vi "Control_stack_solenoid_top.vi"(0 "Valve On?":bool) -> (2 "s? t:f":errorcluster)   [LabVIEW 2010]
panel:
  in  "Reset":bool
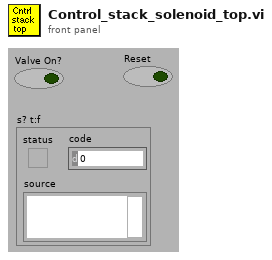
[diagram p1: front panel]
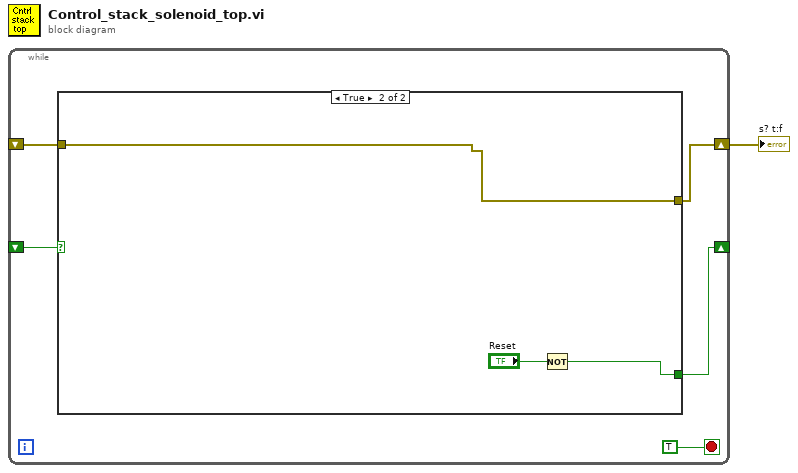
[diagram p0: block diagram]
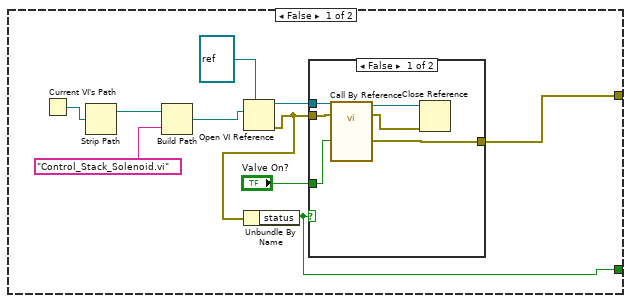
[diagram p2: hidden frame]
diagram:
  n1 = while {
    shift-right: [w5] -> _
    shift-left: _ -> [w6]
    shift-right: [w3] -> w1
    shift-left: _ -> [w2]
    stop <- TRUE stop-if-true
    n2 = case shown="True" w6 {
      tunnel: [w8 w24] -> w5
      tunnel: [w7 w26] -> w3
      tunnel: w2 -> [_ w26]
      frame False {
        n3 = Current VI's Path() -> (path=w16:path)
        n4 = Strip Path(path=w16) -> (stripped path=w15:path)  [unwired: 1 out]
        n5 = Build Path(base path=w15, name or relative path="Control_Stack_Solenoid.vi") -> (appended path=w13:path)
        n6 = Open VI Reference(type specifier VI Refnum (for type only)=refnum<vi> refnum, vi path=w13) -> (vi reference=w11:refnum<vi>, error out=w10:errorcluster)  [unwired: 1 in, 3 out]
        n7 = Unbundle By Name(w10) -> ("status"=w8:bool)
        n8 = case shown="False" w8 {
          tunnel: w11 -> [w22 _]
          tunnel: w10 -> [w21 w23]
          tunnel: [w20 w23] -> w7
          tunnel: "Valve On?" -> [w17 _]
          frame False {
            n9 = call-by-ref "?"(reference=w22, error in=w21, "Valve On?"=w17) -> (reference out=w19:refnum<vi>, error out=w18:errorcluster, "s? t:f"=w20:errorcluster)
            n10 = Close Reference(reference=w19, error in (no error)=w18) -> ()  [unwired: 1 out]
          }
          frame True {
          }
        }
      }
      frame True {
        n11 = Not(x="Reset") -> (.not. x?=w24:bool)
      }
    }
  }
  "s? t:f" <- w1
